vi "tx poulse host_get_IQ_from_fpga.vi"() -> ()   [LabVIEW 2021]
uses:
  <instrlib>/niUsrpRio/Config/v1/Host/Private/LO Source.ctl
  <vilib>/FPGAPlugInAG/USRP 294xR; 295xR 200 MSps/niLvFpga_Open_USRP 294xR; 295xR 200 MSps.vi
  <vilib>/rvi/interface/common/dynamic/niFpgaDynamicAddResources.vi
  <vilib>/rvi/interface/common/niFpgaWaitOnOcc.vi
  <vilib>/Utility/error.llb/Error Cluster From Error Code.vi
  <vilib>/rvi/errors/niLvFpgaAdjustHostInterfaceError.vi
  <vilib>/FPGAPlugInAG/Dynamic/niLvFpga_Close_Dynamic.vi
  <vilib>/rvi/interface/nirviOpenFPGA/nirviOpenFPGA.xnode
  FPGA Bitfiles/Tx_pulse_to_iq_host.lvbitx
  <vilib>/rvi/interface/nirviMethod/nirviMethod.xnode
  <vilib>/rvi/interface/nirviReadWriteControl/nirviReadWriteControl.xnode
  <vilib>/rvi/interface/nirviCloseFPGA/nirviCloseFPGA.xnode
  <instrlib>/niUsrpRio/Config/v1/Host/niUsrpRio Config v1 Host.lvlib
  NiFpgaLv.dll
  <vilib>/rvi/interface/Simulation/niFpgaSimulationCallBeginRW.vi
  <vilib>/rvi/errors/niLvFpgaMergeErrorWithErrorCode.vi
  <vilib>/FPGAPlugInAG/Dynamic/niLvFpga_WriteFifo_Dynamic.vi
  <vilib>/FPGAPlugInAG/Dynamic/niLvFpga_ConfigureFifo_Dynamic.vi
  <vilib>/FPGAPlugInAG/Dynamic/niLvFpga_ReadFifo_Dynamic.vi
panel:
  in  "stop 2":bool
  in  "dcimator":u8
  in  "output file path":path=path "C:/Users/NI/Documents/chaim/chaim_rx/chaim_data/IQ.tdms"
  out "tx free":bool[](array[boolean])=[FALSE, FALSE, FALSE, FALSE, FALSE, FALSE, TRUE, TRUE, TRUE, TRUE, TRUE, TRUE, TRUE, TRUE, TRUE, TRUE]
  out "# pulse sent to FPGA":dbl=22448.0
  out "pulse Tx by FPGA":u32=6287
  out "fpga clock":dbl=13.996499525
  in  "tdms pulse istraction file path":path=path "C:/Users/NI/Documents/chaim/chaim_rx/chaim_data/pulses.tdms"
  in  "stop":bool
  in  "gain 0":dbl=-20.0 format="%#_6p"
  in  "Tx. frequency 0":dbl=2000000000.0 format="%#_6p"
  # "pulse transmitter"
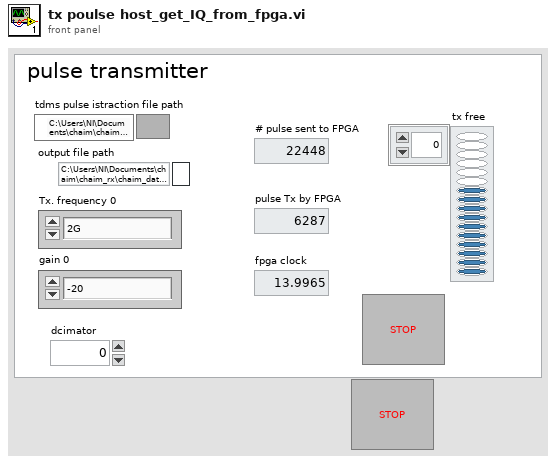
[diagram p1: front panel]
types:
  T1 = enum16{"open", "open or create", "create or replace", "create", "open (read-only)"}
  T2 = typedef "niUsrpRio Config v1 Host.lvlib/LO Source.ctl" = enum16{"Internal", "Companion", "External", "Reimport"}
  T3 = typedef "niUsrpRio Config v1 Host.lvlib/niUsrpRio Session.ctl" = cluster{"FPGA Interface":refnum<k20>, "RIO Interface Number":u32, "Data Clock Rate":u32, "FPGA Data Clock Rate":u32, "Global Settings Register Bus":T4, "Radio 0 Settings Register Bus":T4, "Radio 1 Settings Register Bus":T4, "Radio Settings Bus Semaphore":T5, "DB Queues":T6[], "Characterization Data Valid?":bool, "EEPROM Header":T7, "Device Data Header":T8, "EEPROM Characterization Header":T9, "Characterization Data":T10[], "FPGA Current Version":u32, "FPGA Oldest Compatible Version":u32, "Fixed Logic Current Version":u32, "Fixed Logic Oldest Compatible Version":u32, "FPGA Radio Settings Bus Current Version":u32, "FPGA Radio Settings Bus Oldest Compatible Version":u32, "FPGA Board Config Current Version":u32, "FPGA Board Config Oldest Compatible Version":u32, "Daughterboard Clock Rate":u32, "daughterboard configuration session handles":u64[]}
  T4 = typedef "niInstr Register Bus v0 Host.lvlib/Register Bus Session.ctl" = refnum<queue>
  T5 = typedef "Semaphore RefNum" = refnum<k1>
  T6 = typedef "niUsrpRio Config v1 Host.lvlib/DB Queue Reference.ctl" = refnum<queue>
  T7 = typedef "niUsrpRio Config v1 Host.lvlib/EEPROM Header.ctl" = cluster{"Checksum":u32, "Product Code":u16, "Hardware Current Version":u16, "Hardware Oldest Compatible Version":u16, "EEPROM Map Current Version":u16, "EEPROM Map Oldest Compatible Version":u16, "User Password":string, "Pointer to Factory Header":u32, "Pointer to User Header":u32, "Recommended Interval":u16, "Number of Reserved Bytes":i32, "Number of Daughterboards":u8, "Daughterboard IDs":u16[], "Daughterboard Serial Numbers":string[]}
  T8 = typedef "niUsrpRio Config v1 Host.lvlib/EEPROM Device Data Header.ctl" = cluster{"Checksum":u32, "Number of Channels":u8, "Number of Gain Settings":u16[], "Pointer to Characterization Data":u32[], "Number of Reserved Bytes":i32, "Number of Frequencies":u16[]}
  T9 = typedef "niUsrpRio Config v1 Host.lvlib/EEPROM Characterization Header.ctl" = cluster{"Checksum":u32, "Date":timestamp, "Temperature":sgl, "Misc. Info":string, "Pointer to Device Data Header":u32, "Number of Reserved Bytes":i32}
  T10 = typedef "niUsrpRio Config v1 Host.lvlib/Characterization Data.ctl" = cluster{"Gains[dB]":dbl[], "Frequencies [Hz]":dbl[], "IQ Imbalance Table":T11[], "Measured Gains[dB]":dbl[][]}
  T11 = typedef "niUsrpRio Config v1 Host.lvlib/IQ Imbalance.ctl" = cluster{"Gain Imbalance [linear]":dbl, "Phase Imbalance [radians]":dbl, "Offset":cdb}
  T12 = cluster{"gain I":fxp<+/-,24,3>, "gain Q":fxp<+/-,24,3>}
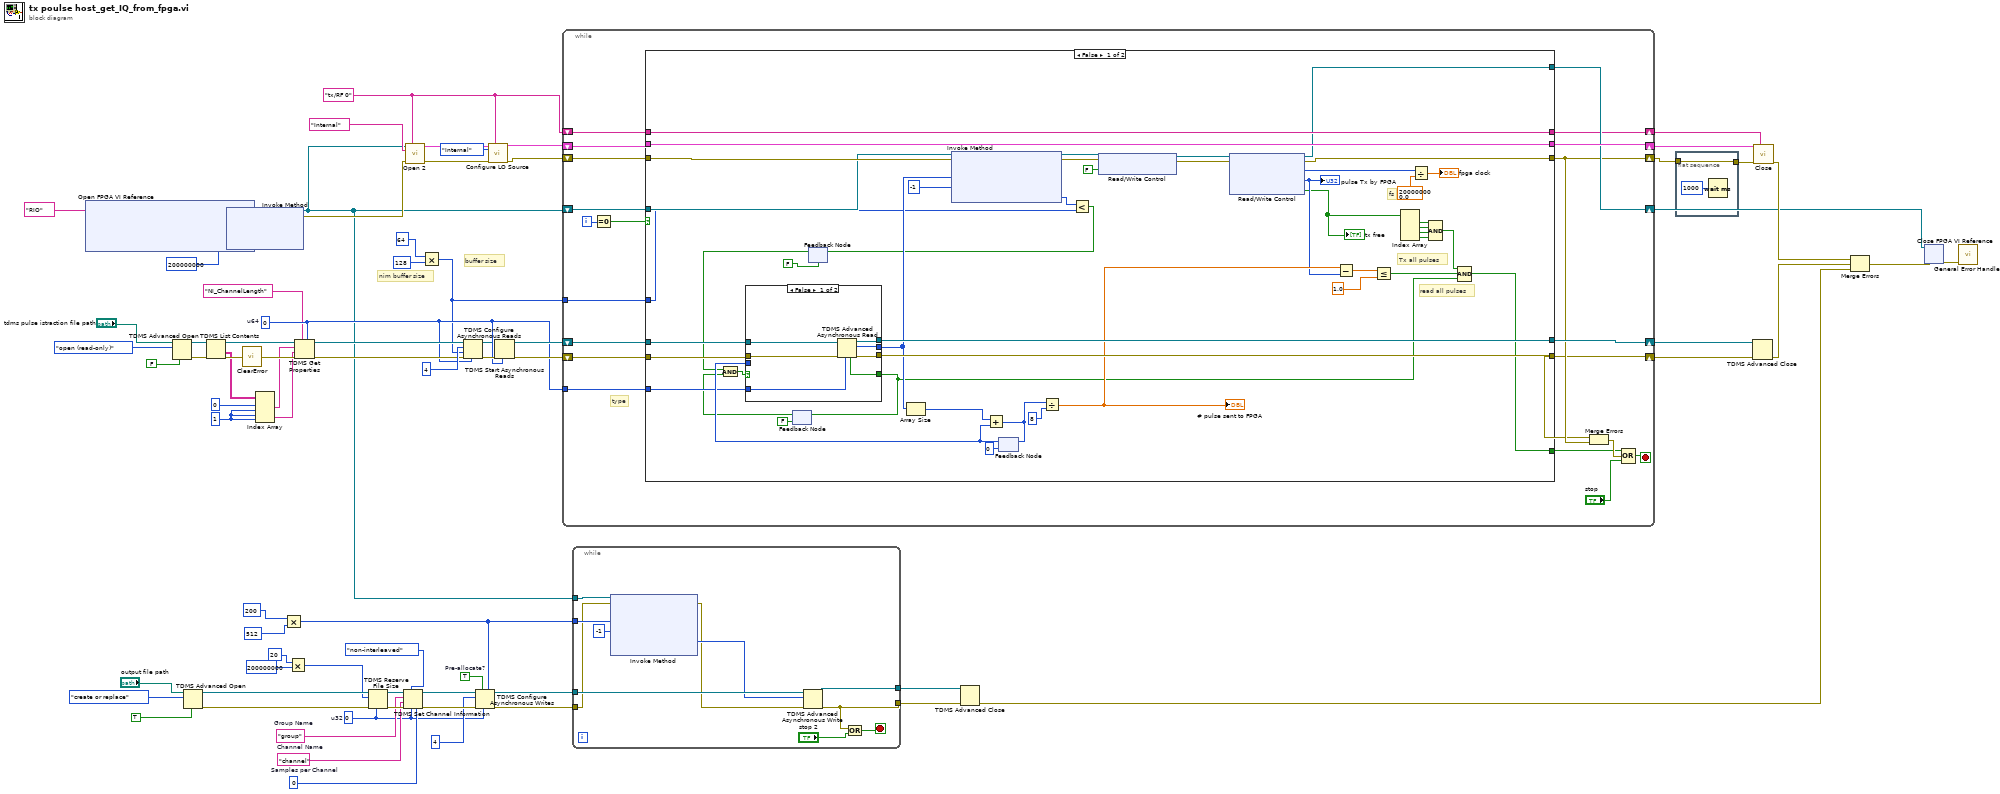
[diagram p0: block diagram]
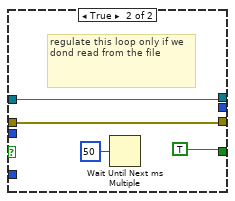
[diagram p2: hidden frame]
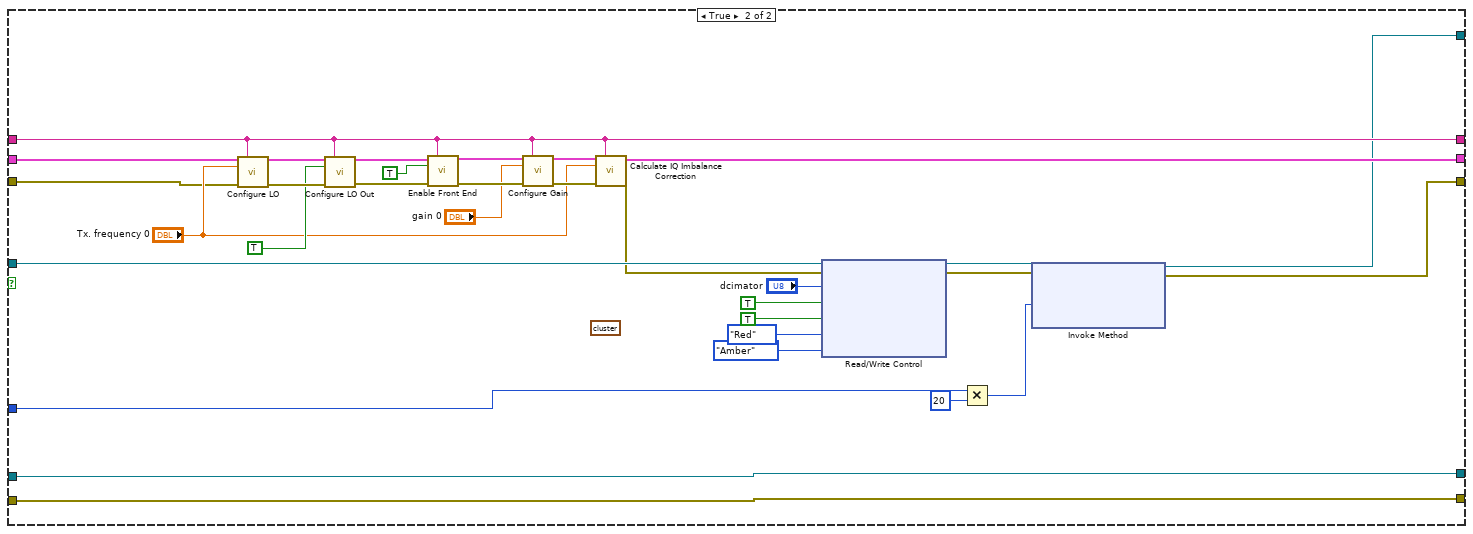
[diagram p3: hidden frame]
diagram:
  w16 = TRUE  # Pre-allocate?
  w19 = "group"  # Group Name
  w20 = "channel"  # Channel Name
  w17 = u32 0  # u32
  w28 = u32 0  # Samples per Channel
  w46 = 1 ("disabled index (col)")
  w42 = u64 0  # u64
  w73 = "tx/RF 0" ("scope")
  # "buffer size"
  # "nim buffer size"
  n1 = xnode ("Open FPGA VI Reference")("resource name"=tag "RIO") -> ("FPGA VI Reference Out"=w32:refnum<k20>, "error out"=w31:errorcluster)  [unwired: 1 in]
  n2 = TDMS Advanced Open(6:FALSE ("Disable Buffering? (T)"), 10:T1."open (read-only)" ("Operation"), 11:"tdms pulse istraction file path") -> (0:w56:errorcluster, 3:w49:refnum<k34>)  [unwired: 2 in, 1 out]
  n3 = TDMS Advanced Open(6:TRUE ("Disable Buffering? (T)"), 10:T1."create or replace" ("operation (0:open)"), 11:"output file path") -> (0:w26:errorcluster, 3:w24:refnum<k34>)  [unwired: 2 in, 1 out]
  n4 = TDMS List Contents(4:w56, 7:w49) -> (0:w54:errorcluster, 1:w45:string[][], 3:w50:refnum<k34>)  [unwired: 1 in, 1 out]
  n5 = xnode "Invoke Method"("FPGA VI Reference In"=w32, "error in"=w31, "Requested Depth"=u32 200000000) -> ("FPGA VI Reference Out"=w10:refnum<k20>, "error out"=w30:errorcluster)  [unwired: 1 out]
  n6 = call <vilib>:"ClearError.vi"("error in (no error)"=w54) -> ("error out"=w57:errorcluster)
  n7 = Index Array(array=w45, index (row) #1=0 ("index (row)"), index (col) #1=w46, index (row) #2=w46, index (col) #2=w46) -> (element #1=w44:string, element #2=w43:string)
  n8 = Multiply(x=u32 200 ("max write size"), y=u32 512 ("max write size")) -> (x*y=w9:u32)
  n9 = Multiply(x=u32 20, y=u32 200000000 ("Requested Depth")) -> (x*y=w1:u32)
  n10 = TDMS Get Properties(5:w42, 7:"NI_ChannelLength" ("property name"), 8:w57, 9:w43, 10:w44, 11:w50) -> (0:w55:errorcluster, 3:w48:refnum<k34>)  [unwired: 4 out]
  n11 = TDMS Reserve File Size(6:w17, 8:w26, 10:w1, 11:w24) -> (0:w25:errorcluster, 3:w23:refnum<k34>)  [unwired: 1 in]
  n12 = TDMS Set Channel Information(4:w28, 6:w17, 7:enum16{"non-interleaved", "interleaved"}."non-interleaved" ("data layout (0:non-interleaved)"), 8:w25, 9:w20, 10:w19, 11:w23) -> (0:w27:errorcluster, 3:w22:refnum<k34>)
  n13 = call <instrlib>:"Open 2.vi"("fpga ref"=w10, "scope"=w73, "Reference Frequency Source"="Internal", "error in"=w30) -> ("niUsrpRio Session (out)"=w65:T3, "error out"=w75:errorcluster)  [unwired: 10 in]
  n14 = Multiply(x=u32 64, y=u32 128 ("buffer size")) -> (x*y=w36:u32)
  n15 = TDMS Configure Asynchronous Reads(6:w42, 8:w55, 9:w36, 10:u32 4 ("Number of Buffers (4)"), 11:w48) -> (0:w59:errorcluster, 3:w41:refnum<k34>)  [unwired: 1 in]
  n16 = TDMS Configure Asynchronous Writes(5:w9, 6:w17, 7:w16, 8:w27, 10:u32 4 ("Max Asynchronous Writes (4)"), 11:w22) -> (0:w7:errorcluster, 3:w8:refnum<k34>)  [unwired: 1 in]
  n17 = call <instrlib>:"Configure LO Source.vi"("niUsrpRio Session"=w65, "scope"=w73, "lo source"=LO_Source."Internal", "error in"=w75) -> ("niUsrpRio Session (out)"=w72:T3, "error out"=w71:errorcluster)  [unwired: 10 in]
  n18 = TDMS Start Asynchronous Reads(6:w42, 8:w59, 11:w41) -> (0:w51:errorcluster, 3:w52:refnum<k34>)  [unwired: 1 in]
  n19 = while {
    shift-right: [w82] -> w34
    shift-left: w71 -> [w95]
    shift-right: [w93] -> w70
    shift-left: w72 -> [w96]
    shift-right: [w92] -> w66
    shift-left: w10 -> [w94]
    shift-right: [w90] -> w69
    shift-left: w73 -> [w91]
    shift-right: [w85] -> w64
    shift-left: w52 -> [w87]
    shift-right: [w81] -> w63
    shift-left: w51 -> [w86]
    tunnel: w42 -> [w84]
    tunnel: w36 -> [w83]
    i -> [w88]
    stop <- w78 stop-if-true
    # "type"
    n20 = Equal To 0?(x=w88) -> (x = 0?=w89:bool)
    n21 = case shown="False" w89 {
      tunnel: w96 -> [w142 w174]
      tunnel: w95 -> [w136 w173]
      tunnel: w94 -> [w135 w172]
      tunnel: [w142 w170] -> w93
      tunnel: [w111 w162] -> w92
      tunnel: [w110 w161] -> w82
      tunnel: w91 -> [w143 w169]
      tunnel: [w143 w169] -> w90
      tunnel: w87 -> [w134 w166]
      tunnel: w86 -> [w133 w165]
      tunnel: [w132 w166] -> w85
      tunnel: [w131 w165] -> w81
      tunnel: w84 -> [w125 _]
      tunnel: w83 -> [w122 w160]
      tunnel: [w104 _] -> w77
      frame False {
        # "fs"
        # "read all pulses"
        # "Tx all pulses"
        n22 = feedback #1(FALSE ("end of file?")) -> (w121:bool)
        n23 = feedback #2(FALSE) -> (w120:bool)
        n24 = Compound Arithmetic op=AND(w120, w121) -> (w117:bool)
        n25 = feedback #3(u32 0) -> (w129:u32)
        n26 = case shown="False" w117 {
          tunnel: w134 -> [w150 w154]
          tunnel: w133 -> [w145 w153]
          tunnel: [w149 w154] -> w132
          tunnel: [w146 w153] -> w131
          tunnel: [w147 _] -> w130
          tunnel: [w148 TRUE ("end of file?")] -> w103
          tunnel: w129 -> [_ _]
          tunnel: w125 -> [w144 _]
          frame False {
            n27 = TDMS Advanced Asynchronous Read(6:w144, 8:w145, 11:w150) -> (0:w146:errorcluster, 2:w147:u64[], 3:w149:refnum<k34>, 4:w148:bool)
          }
          frame True {
            # "regulate this loop only if we dond read from the file"
            n28 = Wait Until Next ms Multiple(millisecond multiple=u32 50) -> ()  [unwired: 1 out]
          }
        }
        n29 = feedback-in #1(w103) -> ()
        n30 = Array Size(array=w130) -> (size(s)=w127:i32)
        n31 = xnode ("Invoke Method")("FPGA VI Reference In"=w135, "error in"=w136, "Data"=w130, "Timeout (ms)"=-1) -> ("FPGA VI Reference Out"=w139:refnum<k20>, "error out"=w140:errorcluster, "Empty Elements Remaining"=w123:u32)
        n32 = Add(x=w127, y=w129) -> (x+y=w116:u32)
        n33 = feedback-in #3(w116) -> ()
        n34 = Divide(x=w116, y=u32 8) -> (x/y=w109:dbl)
        "# pulse sent to FPGA" <- w109
        n35 = Less?(x=w123, y=w122) -> (x < y?=w119:bool)
        n36 = feedback-in #2(w119) -> ()
        n37 = xnode ("Read/Write Control")("FPGA VI Reference In"=w139, "error in"=w140, "reset system clock"=FALSE) -> ("FPGA VI Reference Out"=w138:refnum<k20>, "error out"=w137:errorcluster)
        n38 = xnode ("Read/Write Control")("FPGA VI Reference In"=w138, "error in"=w137) -> ("FPGA VI Reference Out"=w111:refnum<k20>, "error out"=w110:errorcluster, "fpga clock"=w113:u64, "pulse transmitted"=w108:u32, "tx free"=w102:bool[])
        "pulse Tx by FPGA" <- w108
        "tx free" <- w102
        n39 = Subtract(x=w109, y=w108) -> (x-y=w107:dbl)
        n40 = Less Or Equal?(x=w107, y=1.0) -> (x <= y?=w105:bool)
        n41 = Index Array(array=w102) -> (element #1=w101:bool, element #2=w100:bool, element #3=w99:bool, element #4=w98:bool)  [unwired: 4 in]
        n42 = Divide(x=w113, y=200000000.0) -> (x/y=→"fpga clock":dbl)
        n43 = Compound Arithmetic op=AND(w101, w100, w99, w98) -> (w97:bool)
        n44 = Compound Arithmetic op=AND(w97, w105, w103) -> (w104:bool)
      }
      frame True {
        (unwired) T12 {"gain I"=1.0, "gain Q"=1.0} ("tx.gain.0")
        n45 = call <instrlib>:"Configure LO.vi"("niUsrpRio Session"=w174, "scope"=w169, "frequency"="Tx. frequency 0", "error in"=w173) -> ("niUsrpRio Session (out)"=w186:T3, "error out"=w185:errorcluster)  [unwired: 8 in, 2 out]
        n46 = call <instrlib>:"Configure LO Out.vi"("niUsrpRio Session"=w186, "scope"=w169, "enable"=TRUE ("enable 0"), "error in"=w185) -> ("niUsrpRio Session (out)"=w183:T3, "error out"=w180:errorcluster)  [unwired: 10 in]
        n47 = call <instrlib>:"Enable Front End.vi"("niUsrpRio Session"=w183, "scope"=w169, "enable"=TRUE ("enable 0 2"), "error in"=w180) -> ("niUsrpRio Session (out)"=w182:T3, "error out"=w181:errorcluster)  [unwired: 10 in]
        n48 = call <instrlib>:"Configure Gain.vi"("niUsrpRio Session"=w182, "scope"=w169, "gain"="gain 0", "error in"=w181) -> ("niUsrpRio Session (out)"=w177:T3, "error out"=w176:errorcluster)  [unwired: 9 in, 1 out]
        n49 = call <instrlib>:"Calculate IQ Imbalance Correction.vi"("niUsrpRio Session"=w177, "scope"=w169, "frequency"="Tx. frequency 0", "error in"=w176) -> ("niUsrpRio Session (out)"=w170:T3, "error out"=w171:errorcluster)  [unwired: 8 in, 2 out]
        n50 = xnode ("Read/Write Control")("FPGA VI Reference In"=w172, "error in"=w171, "dcimator"="dcimator", "reset system clock"=TRUE, "RF 0/Tx/Enable"=TRUE, "LED/RF 0/TX1 RX1"=enum8{"Off", "Green", "Red", "Amber"}."Red", "LED/RF 1/TX1 RX1"=enum8{"Off", "Green", "Red", "Amber"}."Amber") -> ("FPGA VI Reference Out"=w164:refnum<k20>, "error out"=w163:errorcluster)
        n51 = Multiply(x=w160, y=u32 20) -> (x*y=w158:u32)
        n52 = xnode ("Invoke Method")("FPGA VI Reference In"=w164, "error in"=w163, "Requested Depth"=w158) -> ("FPGA VI Reference Out"=w162:refnum<k20>, "error out"=w161:errorcluster)  [unwired: 1 out]
      }
    }
    n53 = Merge Errors(w81, w82) -> (w79:errorcluster)
    n54 = Compound Arithmetic op=OR(w77, w79, "stop") -> (w78:bool)
  }
  n55 = while {
    tunnel: w10 -> [w197]
    tunnel: w9 -> [w196]
    tunnel: w8 -> [w194]
    tunnel: w7 -> [w191]
    tunnel: [w187] -> w6
    tunnel: [w192] -> w5
    stop <- w188 stop-if-true
    n56 = xnode "Invoke Method"("FPGA VI Reference In"=w197, "error in"=w191, "Number of Elements"=w196, "Timeout (ms)"=-1) -> ("error out"=w190:errorcluster, "Data"=w193:u32[])  [unwired: 2 out]
    n57 = TDMS Advanced Asynchronous Write(8:w190, 10:w193, 11:w194) -> (0:w187:errorcluster, 3:w192:refnum<k34>)
    n58 = Or(x=w187, y="stop 2") -> (x .or. y?=w188:bool)
  }
  n59 = TDMS Advanced Close(8:w6, 11:w5) -> (0:w4:errorcluster)  [unwired: 2 in, 1 out]
  n60 = flat-sequence {
    tunnel: w34 -> [w199]
    tunnel: [w199] -> w33
    frame #0 {
      n61 = Wait (ms)(milliseconds to wait=u32 1000) -> ()  [unwired: 1 out]
    }
  }
  n62 = TDMS Advanced Close(8:w63, 11:w64) -> (0:w62:errorcluster)  [unwired: 2 in, 1 out]
  n63 = call <instrlib>:"Close.vi"("niUsrpRio Session"=w70, "scope"=w69, "error in"=w33) -> ("error out"=w68:errorcluster)  [unwired: 11 in, 1 out]
  n64 = Merge Errors(w68, w62, w4) -> (w67:errorcluster)
  n65 = xnode ("Close FPGA VI Reference")("FPGA VI Reference In"=w66, "error in"=w67) -> ("error out"=w35:errorcluster)
  n66 = call <vilib>:"General Error Handler.vi"("error in (no error)"=w35) -> ()  [unwired: 10 in, 5 out]
